vi "Read XML File content.vi"(8 "error in (no error)":errorcluster, 11 "Path":path) -> (0 "error out":errorcluster, 3 "XML File content":string)   [LabVIEW 2013, in "Modbus System Explorer.lvlib"]
uses:
  Modbus System Explorer.lvlib
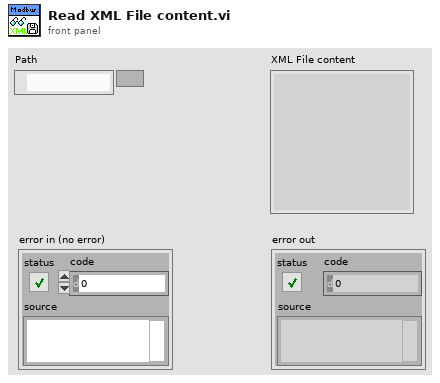
[diagram p1: front panel]
types:
  T1 = enum16{"open", "replace", "create", "open or create", "replace or create", "replace or create with confirmation"}
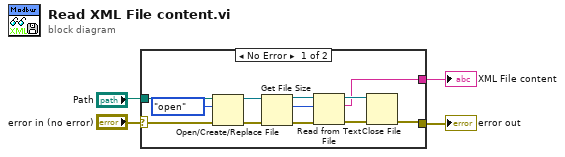
[diagram p0: block diagram]
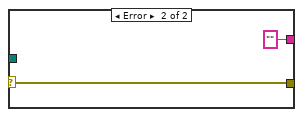
[diagram p2: hidden frame]
diagram:
  n1 = case shown="No Error" "error in (no error)" {
    selector: "error in (no error)" -> [w15 w18]
    tunnel: "Path" -> [w16 _]
    tunnel: [w6 w18] -> w2
    tunnel: [w5 ""] -> w1
    frame No Error {
      n2 = Open/Create/Replace File(file path (use dialog)=w16, error in=w15, operation (0:open)=T1."open") -> (refnum out=w12:refnum<file>, error out=w13:errorcluster)  [unwired: 3 in, 1 out]
      n3 = Get File Size(file=w12, error in=w13) -> (refnum out=w9:refnum<file>, size (in bytes)=w10:i64, 0:w11:errorcluster)
      n4 = Read from Text File(file (use dialog)=w9, count=w10, error in=w11) -> (refnum out=w7:refnum<file>, text=w5:string, error out=w8:errorcluster)  [unwired: 1 in, 1 out]
      n5 = Close File(refnum=w7, error in=w8) -> (error out=w6:errorcluster)  [unwired: 1 out]
    }
    frame Error {
    }
  }
  "error out" <- w2
  "XML File content" <- w1
